vi "Read Actual Position Motor.vi"(8 "error in (no error)":errorcluster, 9 "Axis (1)":i32=1 min=1 max=3, 10 "VISA resource name":refnum<visa-resource-name>, 11 "ESP301 in":refnum<class "ESP301.lvclass">) -> (0 "error out":errorcluster, 1 "Position (units)":dbl format="%.6g", 2 "VISA resource name out":refnum<visa-resource-name>, 3 "ESP301 out":refnum<class "ESP301.lvclass">)   [LabVIEW 2020, in "ESP301.lvclass"]
uses:
  ESP301.lvclass
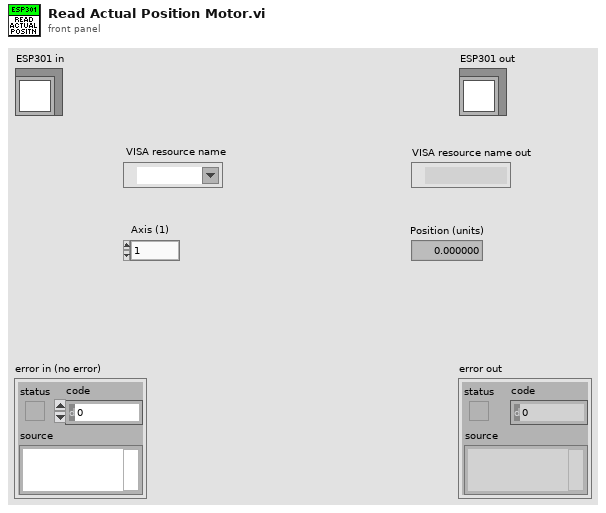
[diagram p1: front panel]
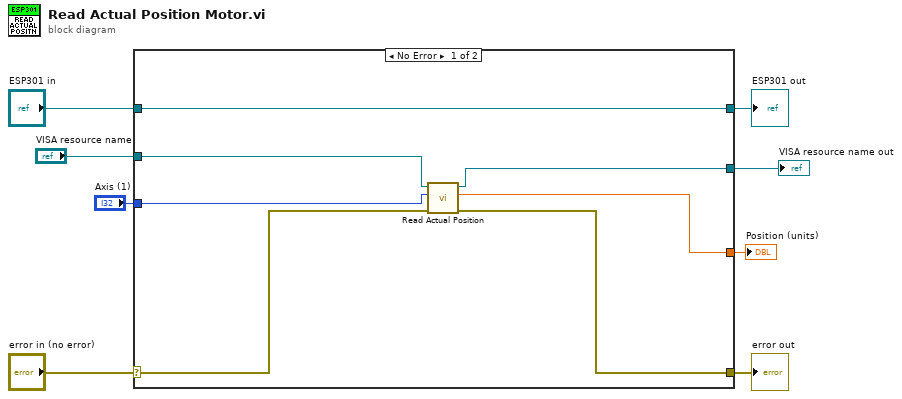
[diagram p0: block diagram]
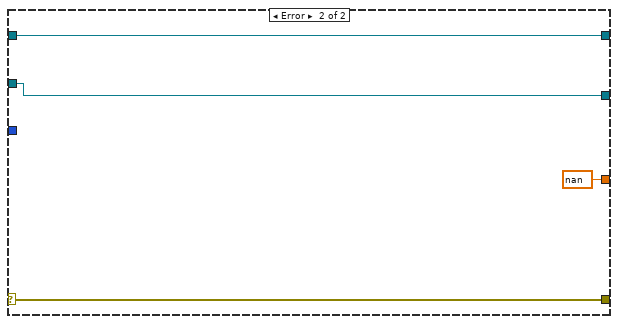
[diagram p2: hidden frame]
diagram:
  n1 = case shown="No Error" "error in (no error)" {
    selector: "error in (no error)" -> [w12 w19]
    tunnel: [w11 w19] -> w7
    tunnel: [w15 w18] -> w5
    tunnel: "ESP301 in" -> [w15 w18]
    tunnel: "VISA resource name" -> [w14 w17]
    tunnel: [w13 w17] -> w3
    tunnel: "Axis (1)" -> [w10 _]
    tunnel: [w9 nan ("Position (units)")] -> w1
    frame No Error {
      n2 = call "Read Actual Position.vi"("error in (no error)"=w12, "Axis (1)"=w10, "VISA resource name"=w14) -> ("error out"=w11:errorcluster, "Position (units)"=w9:dbl, "VISA resource name out"=w13:refnum<visa-resource-name>)  [unwired: 2 in]
    }
    frame Error {
    }
  }
  "error out" <- w7
  "ESP301 out" <- w5
  "VISA resource name out" <- w3
  "Position (units)" <- w1
